vi "mat_transform.vi"(6 "v":dbl, 9 "u":dbl, 10 "Y":sgl, 11 "X":sgl) -> (3 "Real Matrix":T1)   [LabVIEW 2020]
uses:
  <vilib>/Analysis/Matrix/Datatypes/RealMatrix.ctl
  <vilib>/Analysis/Matrix/Numeric/Conversions/Array To Matrix - RA.vi
  <vilib>/Analysis/Matrix/NI_Matrix.lvlib
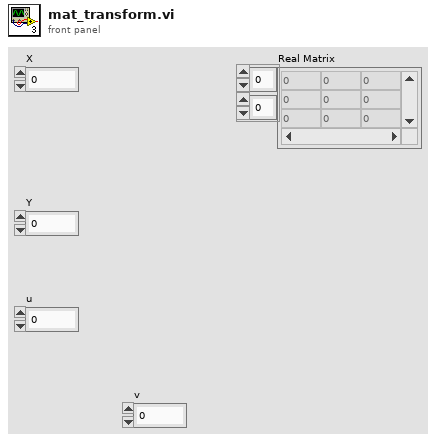
[diagram p1: front panel]
types:
  T1 = typedef "NI_Matrix.lvlib/RealMatrix.ctl" = dbl[][]
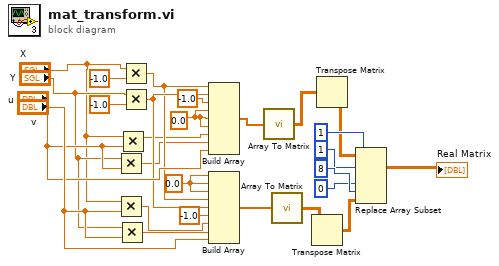
[diagram p0: block diagram]
diagram:
  w11 = 0.0
  w7 = 0.0
  n1 = Multiply(x="Y", y="u") -> (x*y=w10:dbl)
  n2 = Multiply(x="X", y="v") -> (x*y=w18:dbl)
  n3 = Multiply(x="Y", y="v") -> (x*y=w17:dbl)
  n4 = Multiply(x="X", y="u") -> (x*y=w9:dbl)
  n5 = Multiply(x="X", y=-1.0) -> (x*y=w12:dbl)
  n6 = Multiply(x="Y", y=-1.0) -> (x*y=w13:dbl)
  n7 = Build Array(w12, w13, -1.0 ("element"), w7, w7, w7, w9, w10, "u") -> (w26:dbl[])
  n8 = Build Array(w11, w11, w11, w12, w13, -1.0 ("element"), w18, w17, "v") -> (w27:dbl[])
  n9 = call-poly <vilib>:"Array To Matrix.vi"("Real 1D Array"=w26) -> ("Real Matrix (Column Vector)"=w4:T1)
  n10 = call-poly <vilib>:"Array To Matrix.vi"("Real 1D Array"=w27) -> ("Real Matrix (Column Vector)"=w2:T1)
  n11 = Transpose Matrix(1:w2) -> (0:w1:T1)
  n12 = Transpose Matrix(1:w4) -> (0:w3:T1)
  n13 = Replace Array Subset(array=w3, new element=w1, index (dim 0)=1 ("row 1"), index (dim 1)=1 ("row N"), index (dim 2)=0 ("column N"), index (dim 3)=8 ("column 1")) -> (→"Real Matrix":T1)
